vi "test_ccd_GetConfig.vi"(8 "error in":errorcluster, 11 "CCD in":refnum<class "CCD.lvclass">) -> (0 "error out":errorcluster, 3 "CCD out":refnum<class "CCD.lvclass">)   [LabVIEW 2023, in "horiba.test.lvlib"]
uses:
  horiba.test.lvlib
  Classes/CCD/CCD.lvclass
  C:/Projects/Horiba/horiba-labview-sdk/Source/Classes/GenericDevice/GenericDevice.lvclass
  Classes/CCD/SupportedFeatures.ctl
  <vilib>/addons/_JKI Toolkits/Caraya/classes/Assert/Assert Equal Value and Type_Variant.vi
  <vilib>/addons/_JKI Toolkits/Caraya/classes/Test/Test.lvclass
  <vilib>/addons/_JKI Toolkits/Caraya/classes/Assert/Assert.lvclass
  <userlib>/_OpenG.lib/lvdata/lvdata.llb/openg_variant.lvlib
panel:
  # "Connector Pane"
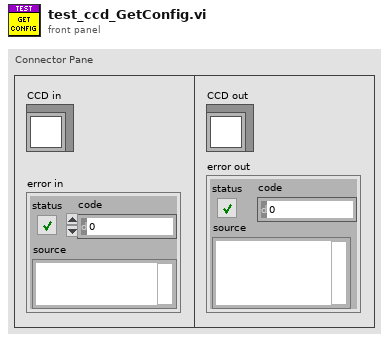
[diagram p1: front panel]
types:
  T1 = typedef "horiba.lvlib/CCD.lvclass/SupportedFeatures.ctl" = cluster{"cf_3PositionSlit":bool, "cf_CMOSOffsetCorrection":bool, "cf_Cleaning":bool, "cf_DSP":bool, "cf_DSPBin2X":bool, "cf_DelayAfterTrigger":bool, "cf_Delays":bool, "cf_EMCCD":bool, "cf_EShutter":bool, "cf_HDR":bool, "cf_Image":bool, "cf_MemorySlots":bool, "cf_Metadata":bool, "cf_MultipleExposeTimes":bool, "cf_MultipleSensors":bool, "cf_PulseSummation":bool, "cf_ROIs":bool, "cf_Signals":bool, "cf_Spectra":bool, "cf_TriggerQualifier":bool, "cf_Triggers":bool}
  T2 = typedef "horiba.lvlib/CCD.lvclass/GetConfig.ctl" = cluster{"centerWavelength":dbl, "chipHSpacing":dbl, "chipHeight":dbl, "chipName":string, "chipSerialNumber":string, "chipVSpacing":dbl, "chipWidth":dbl, "deviceType":string, "fitParameters":dbl[], "gains":T3[], "hardwareAvgAvailable":bool, "lineScan":bool, "productId":string, "serialNumber":string, "signals":T4[], "speeds":T7[], "supportedFeatures":T1, "triggers":T8[], "version":string}
  T3 = typedef "horiba.lvlib/CCD.lvclass/Gain.ctl" = cluster{"info":string, "token":i32}
  T4 = typedef "horiba.lvlib/CCD.lvclass/Signal.ctl" = cluster{"events":T5[], "name":string, "token":i32}
  T5 = typedef "horiba.lvlib/CCD.lvclass/Event.ctl" = cluster{"name":string, "token":i32, "types":T6[]}
  T6 = typedef "horiba.lvlib/CCD.lvclass/Type.ctl" = cluster{"name":string, "token":i32}
  T7 = typedef "horiba.lvlib/CCD.lvclass/Speed.ctl" = cluster{"info":string, "token":i32}
  T8 = typedef "horiba.lvlib/CCD.lvclass/Trigger.ctl" = cluster{"events":T5[], "name":string, "token":i32}
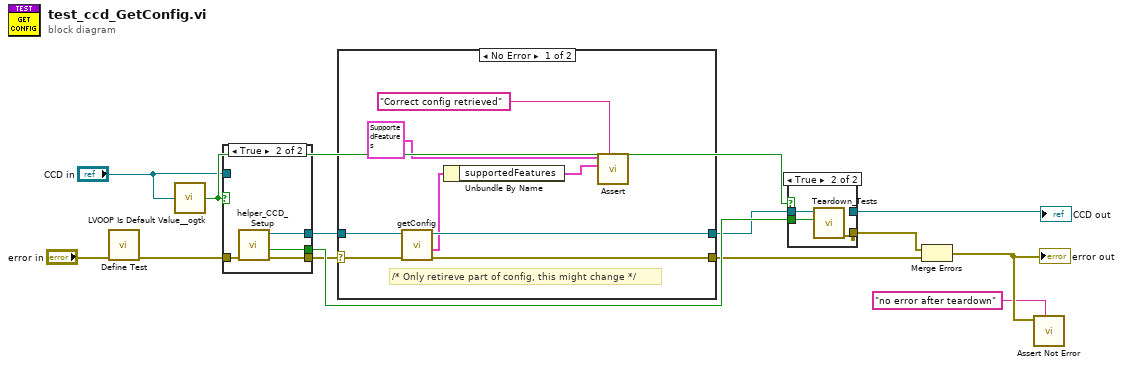
[diagram p0: block diagram]
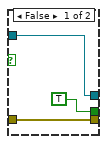
[diagram p3: hidden frame]
diagram:
  n1 = call <vilib>:"Define Test.vi"("error in (no error)"="error in") -> ("error out"=w8:errorcluster)  [unwired: 9 in, 1 out]
  n2 = call <userlib>:"LVOOP Is Default Value__ogtk.vi"("Object"="CCD in") -> ("Is Default Value?"=w9:bool)
  n3 = case shown="True" w9 {
    tunnel: w8 -> [w15 w20]
    tunnel: [w15 w19] -> w4
    tunnel: [w16 w18] -> w6
    tunnel: [TRUE ("Module Was Already Running?") w17] -> w10
    tunnel: "CCD in" -> [w16 _]
    frame False {
    }
    frame True {
      n4 = call "helper_CCD_Setup.vi"("error in"=w20) -> ("error out"=w19:errorcluster, "Module Was Already Running?"=w17:bool, "CCD out"=w18:refnum<class "CCD.lvclass">)  [unwired: 7 in, 1 out]
    }
  }
  n5 = case shown="No Error" w4 {
    selector: w4 -> [w27 w30]
    tunnel: [w24 w29] -> w5
    tunnel: w6 -> [w28 w29]
    tunnel: [w25 w30] -> w3
    frame No Error {
      # "/* Only retireve part of config, this might change */"
      n6 = call "getConfig.vi"("error in (no error)"=w27, "CCD in"=w28) -> ("error out"=w25:errorcluster, "config data"=w23:T2, "CCD out"=w24:refnum<class "CCD.lvclass">)  [unwired: 6 in, 1 out]
      n7 = Unbundle By Name(w23) -> ("supportedFeatures"=w21:T1)
      n8 = call-poly <vilib>:"Assert.vi"("Label"="Correct config retrieved", "Y"=w21, "X"=T1 {"cf_3PositionSlit"=FALSE, "cf_CMOSOffsetCorrection"=FALSE, "cf_Cleaning"=TRUE, "cf_DSP"=FALSE, "cf_DSPBin2X"=FALSE, "cf_DelayAfterTrigger"=FALSE, "cf_Delays"=FALSE, "cf_EMCCD"=FALSE, "cf_EShutter"=FALSE, "cf_HDR"=FALSE, "cf_Image"=TRUE, "cf_MemorySlots"=TRUE, "cf_Metadata"=FALSE, "cf_MultipleExposeTimes"=FALSE, "cf_MultipleSensors"=FALSE, "cf_PulseSummation"=FALSE, "cf_ROIs"=TRUE, "cf_Signals"=TRUE, "cf_Spectra"=TRUE, "cf_TriggerQualifier"=FALSE, "cf_Triggers"=TRUE} ("supportedFeatures")) -> ()  [unwired: 7 in, 2 out]
    }
    frame Error {
    }
  }
  n9 = case shown="True" w9 {
    tunnel: w5 -> [w31 w34]
    tunnel: [_ w33] -> w7
    tunnel: w10 -> [_ w32]
    tunnel: [w31 _] -> w1
    frame False {
    }
    frame True {
      n10 = call "Teardown_Tests.vi"("Module Was Already Running?"=w32, "horiba.lvlib:GenericDevice"=w34) -> ("error out"=w33:errorcluster)  [unwired: 8 in, 1 out]
    }
  }
  "CCD out" <- w1
  n11 = Merge Errors(w7, w3) -> (w12:errorcluster)
  "error out" <- w12
  n12 = call <vilib>:"Assert Not Error.vi"("Label"="no error after teardown", "Not Error?"=w12) -> ()  [unwired: 8 in, 2 out]
